vi "GT_SetCrdStopDec.vi"(6 "decSmoothStop":dbl, 7 "decAbruptStop":dbl, 10 "crd":i16, 11 "rtn":cluster{"rtn":i16, "Func":string}) -> (2 "crd":i16, 3 "rtn":cluster{"rtn":i16, "Func":string})   [LabVIEW 2014]
uses:
  VC6/gts.dll
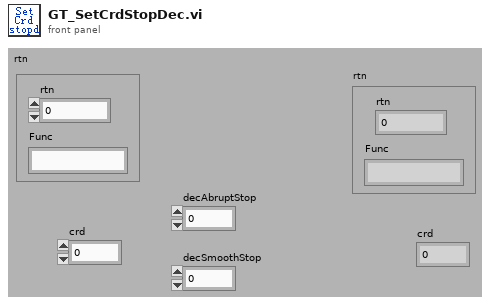
[diagram p1: front panel]
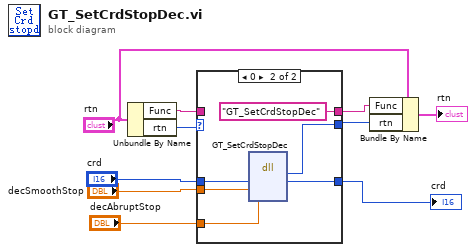
[diagram p0: block diagram]
diagram:
  n1 = Unbundle By Name("rtn") -> ("Func"=w1:string, "rtn"=w6:i16)
  n2 = case shown="0" w6 {
    selector: w6 -> [w13 _]
    tunnel: "crd" -> [w12 w19]
    tunnel: "decSmoothStop" -> [_ w18]
    tunnel: "decAbruptStop" -> [_ w17]
    tunnel: [w12 w16] -> w7
    tunnel: [w13 w15] -> w3
    tunnel: [w11 "GT_SetCrdStopDec" ("Func")] -> w2
    tunnel: w1 -> [w11 _]
    frame Default {
    }
    frame 0 {
      n3 = dll-call lib="PTH2Fabs DNewGTS AC-800LWin7版源程序-20170926gts85VC6gts.dll" fn="GT_SetCrdStopDec"("crd"=w19, "decSmoothStop"=w18, "decAbruptStop"=w17) -> ("rtn"=w15:i16, "crd"=w16:i16)  [unwired: 5 in, 2 out]
    }
  }
  "crd" <- w7
  n4 = Bundle By Name(cluster="rtn", "Func"=w2, "rtn"=w3) -> (→"rtn":cluster{"rtn":i16, "Func":string})
